vi "Configure Step.vi"(0 "VISA resource name":refnum<visa-resource-name>, 5 "Step Component (Frequency)":u16(ring) items=["Step the frequency", "Step the phase", "Step Q / Q high", "Step Q / Q low", "Step CMOS high", "Step CMOS low"], 7 "Step Size (1)":dbl=1.0, 9 "Step Direction (Up)":u16(ring) items=["Up", "Down"], 11 "error in (no error)":errorcluster) -> (4 "VISA resource name out":refnum<visa-resource-name>, 15 "error out":errorcluster)   [LabVIEW 2013, in "Stanford Research CG635.lvlib"]
doc: "<b>Step up/down</b> on the selected component. Will increase\nor decrease the value by the number specified by the step size."
uses:
  <instrlib>/Stanford Research CG635/Stanford Research CG635.lvlib
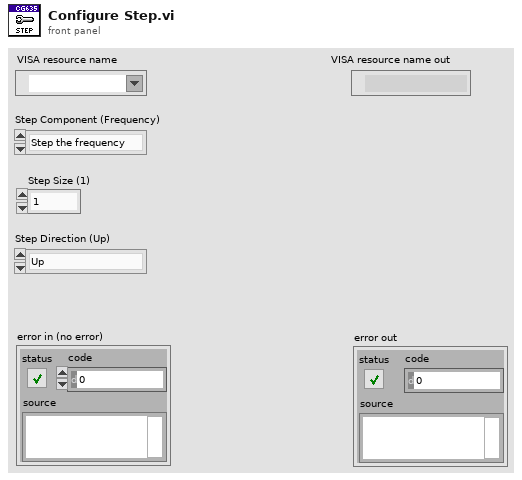
[diagram p1: front panel]
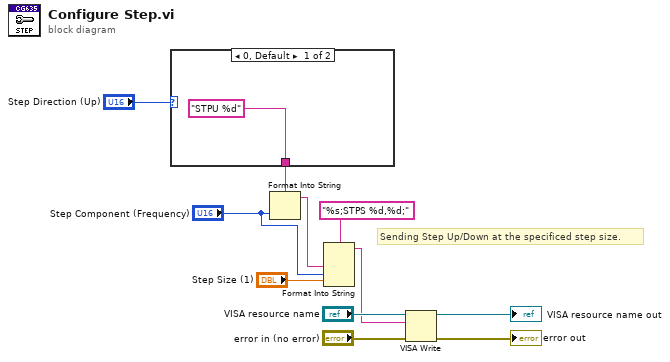
[diagram p0: block diagram]
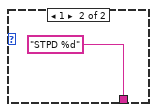
[diagram p2: hidden frame]
diagram:
  # "Sending Step Up/Down at the specificed step size."
  n1 = case shown="0, Default" "Step Direction (Up)" {
    tunnel: ["STPU %d" "STPD %d"] -> w6
    frame 0, Default {
    }
    frame 1 {
    }
  }
  n2 = Format Into String(format string=w6, "Step Component (Frequency)") -> (resulting string=w4:string)  [unwired: 2 in, 1 out]
  n3 = Format Into String(format string="%s;STPS %d,%d;", w4, "Step Component (Frequency)", "Step Size (1)") -> (resulting string=w3:string)  [unwired: 2 in, 1 out]
  n4 = VISA Write(VISA resource name="VISA resource name", write buffer=w3, error in (no error)="error in (no error)") -> (VISA resource name out=→"VISA resource name out":refnum<visa-resource-name>, error out=→"error out":errorcluster)  [unwired: 1 out]
